vi "Auto-Completion On-Off Read 1.vi"(4 "error in (no error)":errorcluster, 6 "Container State":T2, 7 "Display State In":T1) -> (0 "error out":errorcluster, 2 "Value":bool, 3 "Display State Out":T1)   [LabVIEW 2011, in "Intellisense Xcontrol.xctl"]
uses:
  Intellisense Xcontrol.xctl
  <vilib>/_xctls/Container State.ctl
  State 1.ctl
  <vilib>/_xctls/XControlSupport.lvlib
panel:
  # "Replace the Value Indicator below with an Indicator of desired type.\nDo not remove this Indicator or the others from the connector pane. \nDo not change the connector pane pattern.\nThe Value Indicator should always be the second terminal from top on the output side in the connector pane."
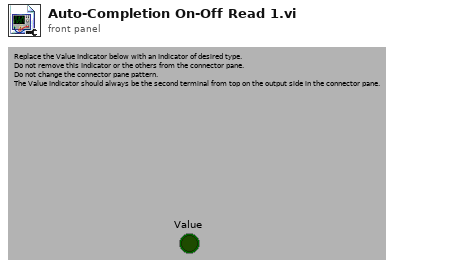
[diagram p1: front panel]
types:
  T1 = typedef "Intellisense Xcontrol.xctl/State 1.ctl" = cluster{"Keyword Array":string[], "Auto-Complete On/Off":bool, "Delimiter":string, "error in (no error)":errorcluster}
  T2 = typedef "XControlSupport.lvlib/Container State.ctl" = cluster{"Indicator?":bool, "Run Mode?":bool, " Refnum":refnum<vi>}
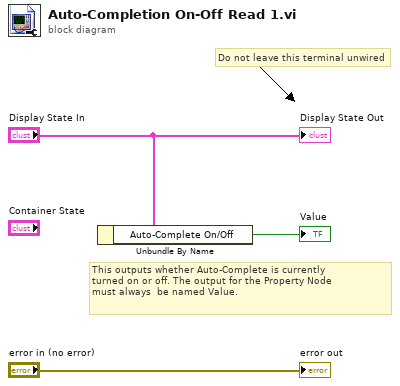
[diagram p0: block diagram]
diagram:
  # "This outputs whether Auto-Complete is currently\nturned on or off. The output for the Property Node\nmust always  be named Value."
  # "Do not leave this terminal unwired"
  n1 = Unbundle By Name("Display State In") -> ("Auto-Complete On/Off"=→"Value":bool)
  "error out" <- "error in (no error)"
  "Display State Out" <- "Display State In"
